vi "Simple Smith Plot.vi"() -> (6 "Pict Out":picture)   [LabVIEW 2012]
doc: "Uses the Smith Plot VI to draw a smith plot in a picture indicator. This example shows how the Smith Plot VIs autoscale the displayed data.\n\nNote: You must have the LabVIEW Full or Professional Development Systems to run this example."
panel:
  in  "New Data":bool=TRUE
  out "Points":cluster{"r":dbl, "x":dbl}[](array[cluster]) {"x" format="%0.2f"; "r" format="%0.2f"}
  in  "Autoscale?":bool=TRUE
  in  "Whole Smith Plot":T1={"x minimum"=-1.0, "x maximum"=1.0, "y minimum"=-1.0, "y maximum"=1.0} {"x minimum" format="%0.2f"; "x maximum" format="%0.2f"; "y minimum" format="%0.2f"; "y maximum" format="%0.2f"}
  in  "Autoscale":T1 {"x minimum" format="%0.2f"; "x maximum" format="%0.2f"; "y minimum" format="%0.2f"; "y maximum" format="%0.2f"}
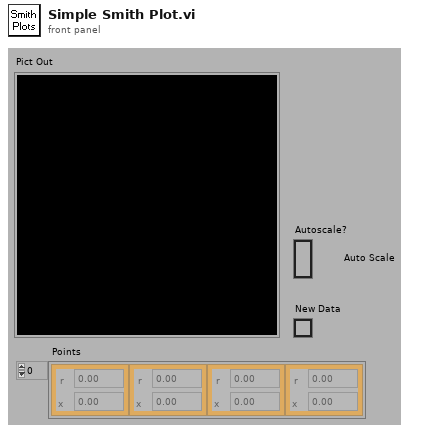
[diagram p1: front panel]
types:
  T1 = cluster{"x minimum":dbl, "x maximum":dbl, "y minimum":dbl, "y maximum":dbl}
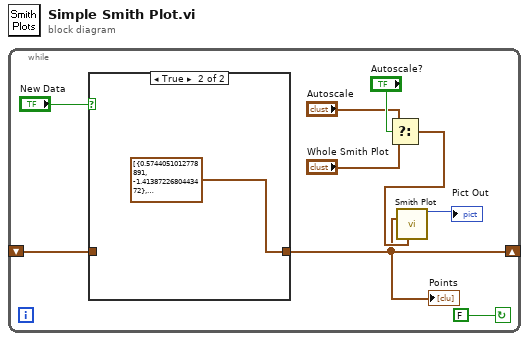
[diagram p0: block diagram]
diagram:
  n1 = while {
    shift-left: _ -> [w2]
    shift-right: [w3] -> _
    stop <- FALSE continue-if-true
    n2 = case shown="True" "New Data" {
      tunnel: [w10 cluster{"r":dbl, "x":dbl}[] [{"r"=0.5744051012778891, "x"=-1.4138722680443472}, {"r"=1.0026691357459314, "x"=2.8699260211341615}] ("Points")] -> w3
      tunnel: w2 -> [w10 _]
      frame False {
      }
      frame True {
      }
    }
    "Points" <- w3
    n3 = Select(t="Autoscale", s="Autoscale?", f="Whole Smith Plot") -> (s? t:f=w8:T1)
    n4 = call <vilib>:"Smith Plot.vi"("smith plot"=w3, "smith plot section"=w8) -> ("new picture"=→"Pict Out":picture)  [unwired: 3 in, 10 out]
  }
